vi "Sort 2D Array.vi"(1 "?":dbl[][](array[numeric]) format="%.2f", 2 "First Column":bool) -> (0 "?":dbl[][](array[numeric]) format="%.2f")   [LabVIEW 2020]
doc: "Sorts a two dimensional array of doubles on the values of the first array.\nScott Hannahs, NHMFL-FSU, June 1995"
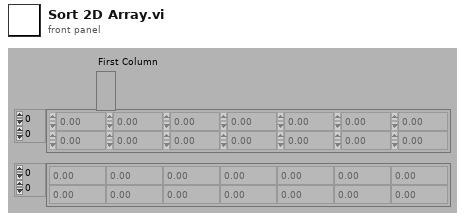
[diagram p1: front panel]
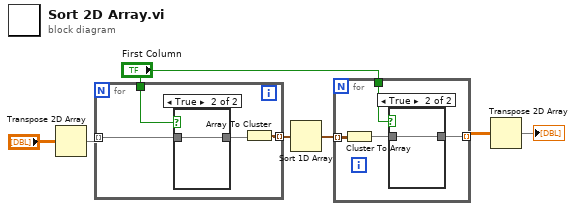
[diagram p0: block diagram]
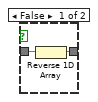
[diagram p2: hidden frame]
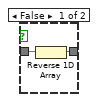
[diagram p3: hidden frame]
diagram:
  n1 = Transpose 2D Array(2D array="?") -> (transposed array=w5:dbl[][])
  n2 = for {
    tunnel: w5 -> [w9] mode=indexing
    tunnel: [w11] -> w3 mode=indexing
    tunnel: "First Column" -> [w8]
    n3 = case shown="True" w8 {
      tunnel: [w13 w14] -> w10
      tunnel: w9 -> [w12 w14]
      frame False {
        n4 = Reverse 1D Array(array=w12) -> (reversed array=w13:dbl[])
      }
      frame True {
      }
    }
    n5 = Array To Cluster(array=w10) -> (cluster=w11:cluster{"[0]":dbl, "[1]":dbl})
  }
  n6 = Sort 1D Array(array=w3) -> (sorted array=w7:cluster{"[0]":dbl, "[1]":dbl}[])
  n7 = for {
    tunnel: w7 -> [w18] mode=indexing
    tunnel: "First Column" -> [w17]
    tunnel: [w16] -> w1 mode=indexing
    n8 = Cluster To Array(cluster=w18) -> (array=w15:dbl[])
    n9 = case shown="True" w17 {
      tunnel: [w20 w21] -> w16
      tunnel: w15 -> [w19 w21]
      frame False {
        n10 = Reverse 1D Array(array=w19) -> (reversed array=w20:dbl[])
      }
      frame True {
      }
    }
  }
  n11 = Transpose 2D Array(2D array=w1) -> (transposed array=→"?":dbl[][])
